vi "DMD Controller v1.3_master_mode.vi"() -> ()   [LabVIEW 2018]
uses:
  Program Files (x86)/National Instruments/LabVIEW 2012/user.lib/alpV42 X86/alpV42 X86.lvlib
panel:
  out "Load number":i32
  out "function return":i32
  in  "停止":bool
  in  "Pattern 路径":path=path "T:/SequenceTextAndCircle-XGA"
  out "SequenceIdPtr out":u32
  in  "PicNum":i32=10
  out "UserVarPtr out":i32
  # "DMD 刺激程序 V1.3\n退出时点击程序的停止按钮, \n不要点击LabVIEW的退出按钮"
  # "(文件名字必须是1 2 ... 50.png)"
  # "'0'"
  # "'1'"
  # "'7980'"
  # "= PicNum - 1"
  # "注意: 出现任何与  '红色信息不符的序列号'   证明有问题 !!!   请检查 !!"
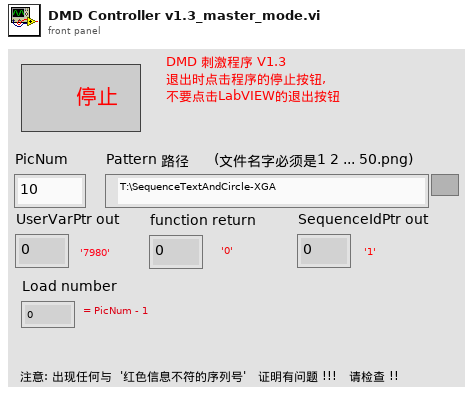
[diagram p1: front panel]
types:
  T1 = typedef "imagedata.ctl" = cluster{"image type":i32, "image depth":i32, "image":u8[], "mask":u8[], "colors":u32[], "Rectangle":cluster{"left":i16, "top":i16, "right":i16, "bottom":i16}}
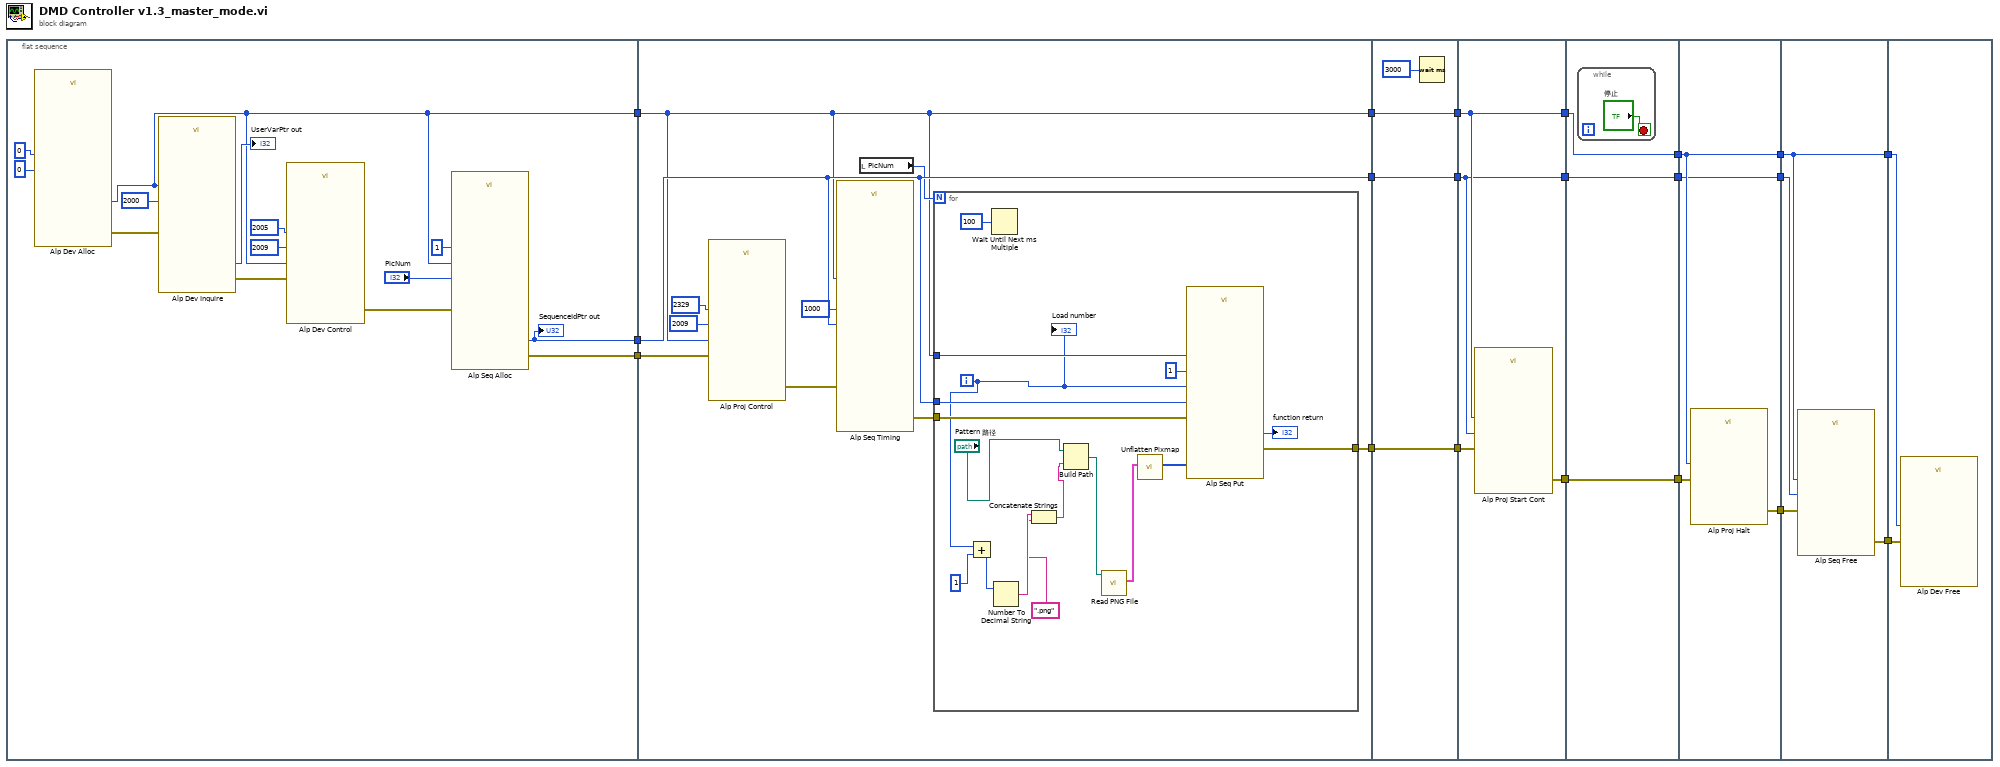
[diagram p0: block diagram]
diagram:
  n1 = flat-sequence {
    tunnel: [w22] -> w20
    tunnel: [w28] -> w16
    tunnel: [w25] -> w7
    tunnel: w20 -> [w37]
    tunnel: [w37] -> w11
    tunnel: w16 -> [w42]
    tunnel: [w42] -> w9
    tunnel: w7 -> [w40]
    tunnel: [w38] -> w6
    tunnel: w11 -> [w65]
    tunnel: [w65] -> w10
    tunnel: w9 -> [w64]
    tunnel: [w64] -> w8
    tunnel: w6 -> [w62]
    tunnel: [w62] -> w5
    tunnel: w10 -> [w69]
    tunnel: [w69] -> w19
    tunnel: w8 -> [w68]
    tunnel: [w68] -> w15
    tunnel: w5 -> [w67]
    tunnel: [w66] -> w3
    tunnel: w19 -> [w72]
    tunnel: [w72] -> w18
    tunnel: w15 -> [w71]
    tunnel: [w71] -> w14
    tunnel: [w70] -> w4
    tunnel: w3 -> [w70]
    tunnel: w18 -> [w77]
    tunnel: [w77] -> w17
    tunnel: w14 -> [w76]
    tunnel: [w76] -> w13
    tunnel: w4 -> [w75]
    tunnel: [w74] -> w2
    tunnel: w17 -> [w80]
    tunnel: w13 -> [w81]
    tunnel: [w80] -> w12
    tunnel: w2 -> [w79]
    tunnel: [w78] -> w1
    tunnel: w12 -> [w83]
    tunnel: w1 -> [w82]
    frame #0 {
      n2 = call "Alp Dev Alloc.vi"("InitFlag"=0, "DeviceNum"=0) -> ("error out"=w27:errorcluster, "DeviceIdPtr out"=w22:u32)  [unwired: 7 in, 1 out]
      n3 = call "Alp Dev Inquire.vi"("error in (no error)"=w27, "InquireType"=2000, "DeviceId"=w22) -> ("error out"=w26:errorcluster, "UserVarPtr out"=→"UserVarPtr out":i32)  [unwired: 6 in, 1 out]
      n4 = call "Alp Dev Control.vi"("error in (no error)"=w26, "ControlValue"=2009, "ControlType"=2005, "DeviceId"=w22) -> ("error out"=w21:errorcluster)  [unwired: 6 in, 1 out]
      n5 = call "Alp Seq Alloc.vi"("error in (no error)"=w21, "PicNum"="PicNum", "BitPlanes"=1, "DeviceId"=w22) -> ("error out"=w25:errorcluster, "SequenceIdPtr out"=w28:u32)  [unwired: 5 in, 1 out]
      "SequenceIdPtr out" <- w28
    }
    frame #1 {
      n6 = call "Alp Proj Control.vi"("error in (no error)"=w40, "ControlValue"=2009, "ControlType"=2329, "DeviceId"=w37) -> ("error out"=w35:errorcluster)  [unwired: 6 in, 1 out]
      n7 = call "Alp Seq Timing.vi"("PictureTime"=1000, "error in (no error)"=w35, "SequenceId"=w42, "DeviceId"=w37) -> ("error out"=w39:errorcluster)  [unwired: 6 in, 1 out]
      n8 = local read "PicNum"() -> (w41:i32)
      n9 = for {
        N: w41 -> [_]
        tunnel: w42 -> [w61]
        tunnel: w37 -> [w60]
        tunnel: w39 -> [w54]
        tunnel: [w53] -> w38
        i -> [w50]
        n10 = Add(x=w50, y=1) -> (x+y=w48:i32)
        n11 = Wait Until Next ms Multiple(millisecond multiple=u32 100 ("毫秒倍数")) -> ()  [unwired: 1 out]
        n12 = Number To Decimal String(number=w48) -> (decimal integer string=w47:string)  [unwired: 1 in]
        n13 = Concatenate Strings(w47, ".png") -> (w45:string)
        n14 = Build Path(base path="Pattern 路径", name or relative path=w45) -> (appended path=w57:path)
        n15 = call <vilib>:"Read PNG File.vi"("path to PNG file"=w57) -> ("image data"=w59:T1)  [unwired: 8 in, 2 out]
        n16 = call <vilib>:"Unflatten Pixmap.vi"("image data"=w59) -> ("8-bit pixmap"=w56:u8[][])  [unwired: 4 in, 6 out]
        n17 = call "Alp Seq Put.vi"("UserArrayPtr"=w56, "PicLoad"=1, "error in (no error)"=w54, "PicOffset"=w50, "SequenceId"=w61, "DeviceId"=w60) -> ("error out"=w53:errorcluster, "function return"=→"function return":i32)  [unwired: 4 in]
        "Load number" <- w50
      }
    }
    frame #2 {
      n18 = Wait (ms)(milliseconds to wait=u32 3000 ("等待时间（毫秒）")) -> ()  [unwired: 1 out]
    }
    frame #3 {
      n19 = call "Alp Proj Start Cont.vi"("error in (no error)"=w67, "SequenceId"=w68, "DeviceId"=w69) -> ("error out"=w66:errorcluster)  [unwired: 7 in, 1 out]
    }
    frame #4 {
      n20 = while {
        stop <- "停止" stop-if-true
      }
    }
    frame #5 {
      n21 = call "Alp Proj Halt.vi"("error in (no error)"=w75, "DeviceId"=w77) -> ("error out"=w74:errorcluster)  [unwired: 8 in, 1 out]
    }
    frame #6 {
      n22 = call "Alp Seq Free.vi"("error in (no error)"=w79, "SequenceId"=w81, "DeviceId"=w80) -> ("error out"=w78:errorcluster)  [unwired: 7 in, 1 out]
    }
    frame #7 {
      n23 = call "Alp Dev Free.vi"("error in (no error)"=w82, "DeviceId"=w83) -> ()  [unwired: 8 in, 2 out]
    }
  }
